vi "IMGSettings.vi"(8 "error in (no error)":errorcluster caption="错误输入（无错误）", 11 "IMG路径":path) -> (0 "error out":errorcluster caption="错误输出", 1 "type":string, 3 "extension":string caption="extname")   [LabVIEW 2016, in "EPUB.lvclass"]
uses:
  EPUB.lvclass
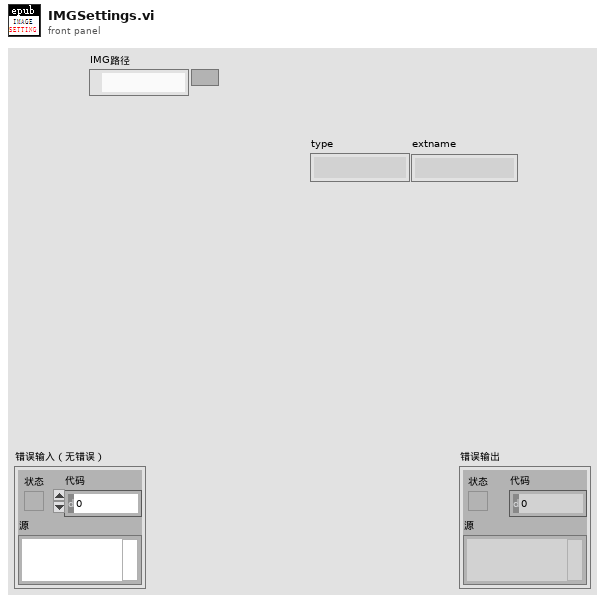
[diagram p1: front panel]
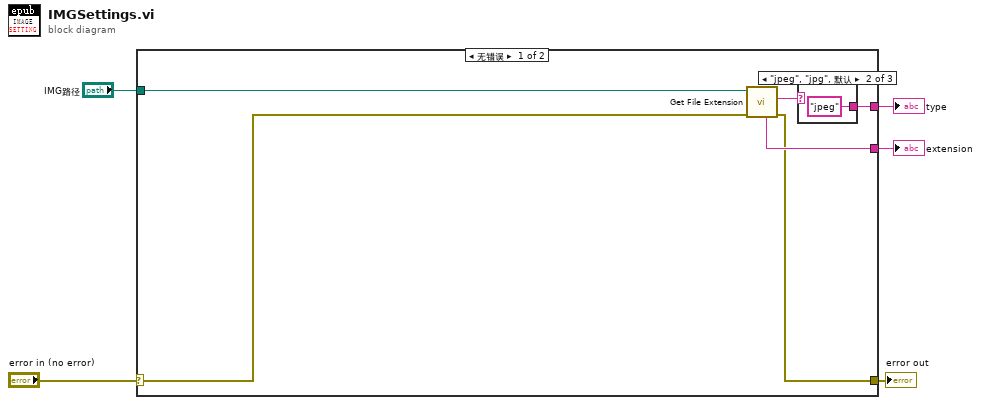
[diagram p0: block diagram]
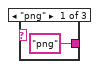
[diagram p2: hidden frame]
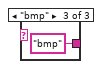
[diagram p3: hidden frame]
diagram:
  n1 = case shown="无错误" "error in (no error)" {
    selector: "error in (no error)" -> [w7 w15]
    tunnel: [w8 w15] -> w4
    tunnel: [w10 _] -> w3
    tunnel: [w9 _] -> w2
    tunnel: "IMG路径" -> [w6 _]
    frame No Error {
      n2 = call <vilib>:"Get File Extension.vi"("error in (no error)"=w7, "file"=w6) -> ("error out"=w8:errorcluster, "lowercase file extension"=w11:string, "unmodified file extension"=w9:string)  [unwired: 5 in, 2 out]
      n3 = case shown="\"jpeg\", \"jpg\", 默认" w11 {
        tunnel: ["png" "jpeg" "bmp"] -> w10
        frame "png" {
        }
        frame "jpeg", "jpg", Default {
        }
        frame "bmp" {
        }
      }
    }
    frame Error {
    }
  }
  "error out" <- w4
  "type" <- w3
  "extension" <- w2
